vi "2DGaussianRotationModel.vi"(3 "output control":T1, 4 "data":T2, 5 "X":dbl[](array[numeric]), 6 "a":dbl[](array[numeric])) -> (0 "error out":errorcluster, 1 "f'(X,a)":dbl[][](array[numeric]), 2 "f(X,a)":dbl[](array[numeric]))   [LabVIEW 2009]
doc: "This template is the starting point for creating a model function to be passed to the Nonlinear Curve Fit.vi."
uses:
  <vilib>/gmath/NumericalOptimization/objective function data.ctl
  <vilib>/gmath/NumericalOptimization/LM_output select.ctl
  <vilib>/Analysis/Matrix/Numeric/Conversions/Array To Matrix - RA2.vi
  <vilib>/Analysis/baseanly.llb/A x Vector.vi
  <vilib>/Analysis/NI_AALBase.lvlib
  <vilib>/Analysis/Matrix/NI_Matrix.lvlib
  <vilib>/gmath/NI_Gmath.lvlib
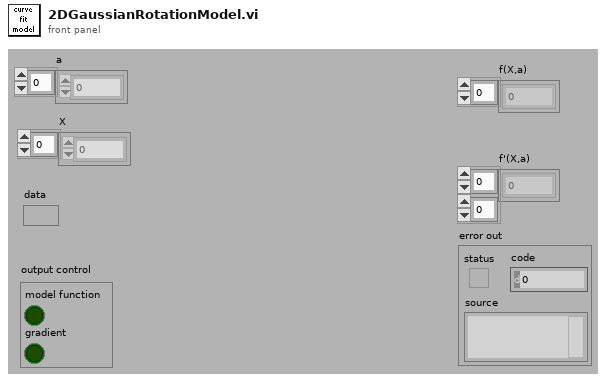
[diagram p1: front panel]
types:
  T1 = typedef "NI_Gmath.lvlib/LM_output select.ctl" = cluster{"model function":bool, "gradient":bool}
  T2 = typedef "NI_Gmath.lvlib/objective function data.ctl" = variant
  T3 = typedef "NI_Matrix.lvlib/RealMatrix.ctl" = dbl[][]
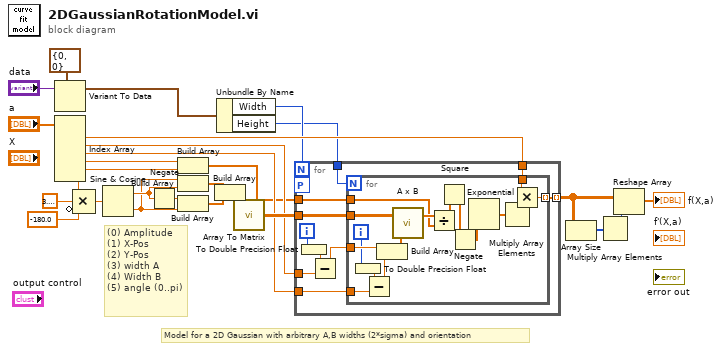
[diagram p0: block diagram]
diagram:
  # "Model for a 2D Gaussian with arbitrary A,B widths (2*sigma) and orientation"
  # "(0) Amplitude\n(1) X-Pos\n(2) Y-Pos\n(3) width A\n(4) Width B\n(5) angle (0..pi)"
  n1 = Variant To Data(Variant="data", type=cluster{"Width":i32, "Height":i32} {"Width"=0, "Height"=0} ("Plot Area:Size")) -> (data=w13:cluster{"Width":i32, "Height":i32})  [unwired: 1 in, 1 out]
  n2 = Index Array(array="a") -> (element #1=w17:dbl, element #2=w7:dbl, element #3=w6:dbl, element #4=w16:dbl, element #5=w15:dbl, element #6=w5:dbl)  [unwired: 6 in]
  n3 = Compound Arithmetic op=MULTIPLY(w5, 3.141592653589793, invert -180.0 ("value")) -> (w4:dbl)
  n4 = Sine & Cosine(0:w4) -> (1:w26:dbl, 2:w25:dbl)
  n5 = Negate(x=w26) -> (-x=w27:dbl)
  n6 = Build Array(w16, w15) -> (w1:dbl[])
  n7 = Build Array(w25, w26) -> (w24:dbl[])
  n8 = Build Array(w27, w25) -> (w23:dbl[])
  n9 = Build Array(w24, w23) -> (w22:dbl[][])
  n10 = Unbundle By Name(w13) -> ("Width"=w9:i32, "Height"=w8:i32)
  n11 = call-poly <vilib>:"Array To Matrix.vi"("Real 2D Array"=w22) -> ("Real Matrix"=w21:T3)
  n12 = for {
    N: w9 -> [_]
    tunnel: w21 -> [w37]
    tunnel: w1 -> [w36]
    tunnel: [w35] -> w20 mode=indexing
    tunnel: w17 -> [w34]
    tunnel: w8 -> [w33]
    tunnel: w7 -> [w30]
    tunnel: w6 -> [w28]
    workers-P: _ -> [_]
    i -> [w32]
    n13 = To Double Precision Float(number=w32) -> (double precision float=w31:dbl)
    n14 = Subtract(x=w31, y=w30) -> (x-y=w29:dbl)
    n15 = for {
      N: w33 -> [_]
      tunnel: w29 -> [w53]
      tunnel: w37 -> [w51]
      tunnel: w36 -> [w49]
      tunnel: [w46] -> w35 mode=indexing
      tunnel: w34 -> [w45]
      tunnel: w28 -> [w42]
      i -> [w44]
      n16 = To Double Precision Float(number=w44) -> (double precision float=w43:dbl)
      n17 = Subtract(x=w43, y=w42) -> (x-y=w41:dbl)
      n18 = Build Array(w53, w41) -> (w52:dbl[])
      n19 = call-poly <vilib>:"A x B.vi"("Vector"=w52, "A"=w51) -> ("A x Vector"=w50:dbl[])  [unwired: 1 out]
      n20 = Divide(x=w50, y=w49) -> (x/y=w40:dbl[])
      n21 = Square(x=w40) -> (x^2=w39:dbl[])
      n22 = Negate(x=w39) -> (-x=w38:dbl[])
      n23 = Exponential(1:w38) -> (0:w48:dbl[])
      n24 = Multiply Array Elements(1:w48) -> (0:w47:dbl)
      n25 = Multiply(x=w45, y=w47) -> (x*y=w46:dbl)
    }
  }
  n26 = Array Size(array=w20) -> (size(s)=w18:i32[])
  n27 = Multiply Array Elements(1:w18) -> (0:w19:i32)
  n28 = Reshape Array(w20, w19) -> (→"f(X,a)":dbl[])
